vi "SLSC Convert Items - String to Variants.vi"(0 "Datatype":string, 5 "Value":string, 9 "Reset Value":string, 12 "enums":T1[](array[typedef]), 13 "string enums":cluster{"name":string, "string enums":string}[](array[cluster])) -> (4 "Value":variant, 6 "Reset Value":variant, 8 "Value (DBL)":dbl, 10 "Reset Value (DBL)":dbl)   [LabVIEW 2017, in "SLSC Tree Control.lvlib"]
doc: "Converts the string values of the tree control to variants and doubles datatypes."
uses:
  SLSC Tree Control.lvlib
  SLSC EDS API/JSON parsing/enum.ctl
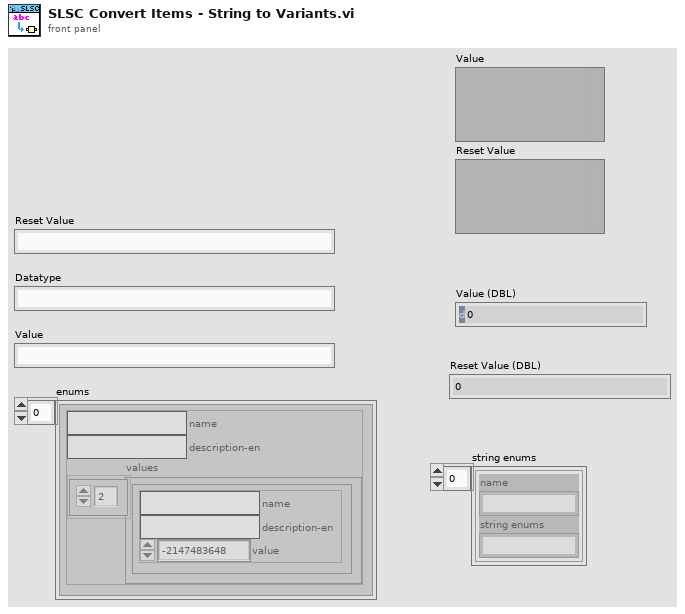
[diagram p1: front panel]
types:
  T1 = typedef "enum.ctl" = cluster{"name":string, "description-en":string, "values":cluster{"name":string, "description-en":string, "value":i32}[]}
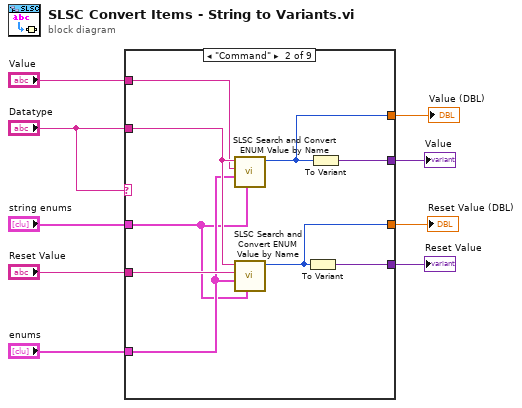
[diagram p0: block diagram]
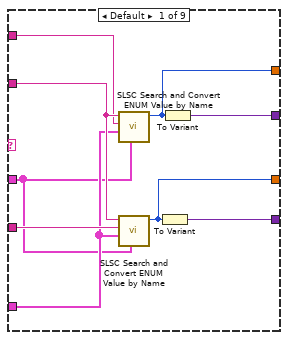
[diagram p2: hidden frame]
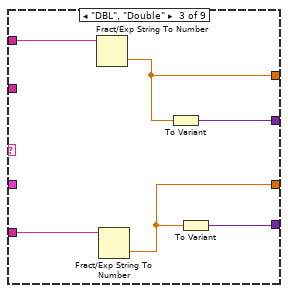
[diagram p3: hidden frame]
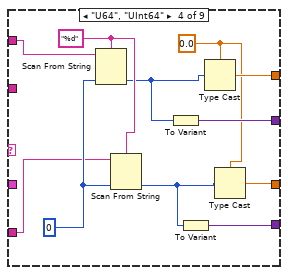
[diagram p4: hidden frame]
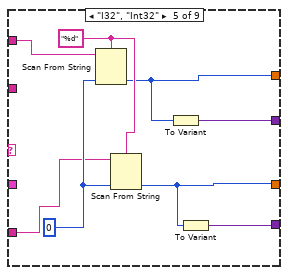
[diagram p5: hidden frame]
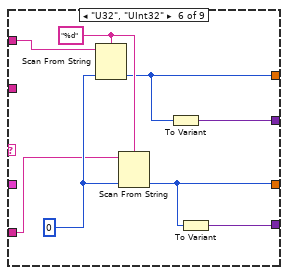
[diagram p6: hidden frame]
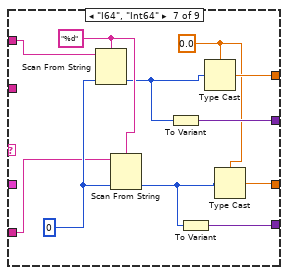
[diagram p7: hidden frame]
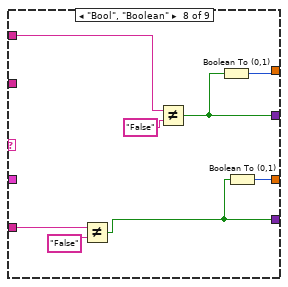
[diagram p8: hidden frame]
diagram:
  n1 = case shown="\"Command\"" "Datatype" {
    tunnel: "Reset Value" -> [w18 w27 w31 w40 w49 w56 w67 w77 _]
    tunnel: "Datatype" -> [w17 w26 _ _ _ _ _ _ _]
    tunnel: "enums" -> [w16 w25 _ _ _ _ _ _ _]
    tunnel: "string enums" -> [w15 w24 _ _ _ _ _ _ _]
    tunnel: "Value" -> [w14 w23 w32 w42 w45 w58 w69 w76 w80]
    tunnel: [w13 w22 w33 w44 w52 w60 w71 w74 w80] -> w4
    tunnel: [w12 w21 w30 w43 w51 w59 w70 w72 _] -> w3
    tunnel: [w11 w20 w29 w37 w47 w54 w64 w75 _] -> w2
    tunnel: [w10 w19 w28 w36 w46 w53 w63 w73 _] -> w1
    frame Default {
      n2 = call "SLSC Search and Convert ENUM Value by Name.vi"("Enum Strings"=w15, "enums"=w16, "Value"=w14, "Datatype Name"=w17) -> ("Value"=w11:i32)  [unwired: 5 in, 2 out]
      n3 = call "SLSC Search and Convert ENUM Value by Name.vi"("Enum Strings"=w15, "enums"=w16, "Value"=w18, "Datatype Name"=w17) -> ("Value"=w10:i32)  [unwired: 5 in, 2 out]
      n4 = To Variant(anything=w10) -> (Variant=w12:variant)
      n5 = To Variant(anything=w11) -> (Variant=w13:variant)
    }
    frame "Command" {
      n6 = call "SLSC Search and Convert ENUM Value by Name.vi"("Enum Strings"=w24, "enums"=w25, "Value"=w23, "Datatype Name"=w26) -> ("Value"=w20:i32)  [unwired: 5 in, 2 out]
      n7 = call "SLSC Search and Convert ENUM Value by Name.vi"("Enum Strings"=w24, "enums"=w25, "Value"=w27, "Datatype Name"=w26) -> ("Value"=w19:i32)  [unwired: 5 in, 2 out]
      n8 = To Variant(anything=w19) -> (Variant=w21:variant)
      n9 = To Variant(anything=w20) -> (Variant=w22:variant)
    }
    frame "DBL", "Double" {
      n10 = Fract/Exp String To Number(string=w32) -> (number=w29:dbl)  [unwired: 3 in, 1 out]
      n11 = Fract/Exp String To Number(string=w31) -> (number=w28:dbl)  [unwired: 3 in, 1 out]
      n12 = To Variant(anything=w29) -> (Variant=w33:variant)
      n13 = To Variant(anything=w28) -> (Variant=w30:variant)
    }
    frame "U64", "UInt64" {
      w34 = 0.0 ("Value")
      w39 = "%d" ("format string")
      w41 = u64 0 ("default (0 U32)")
      n14 = Scan From String(format string=w39, input string=w42, default 1=w41) -> (output 1=w38:u64)  [unwired: 2 in, 3 out]
      n15 = Scan From String(format string=w39, input string=w40, default 1=w41) -> (output 1=w35:u64)  [unwired: 2 in, 3 out]
      n16 = To Variant(anything=w38) -> (Variant=w44:variant)
      n17 = To Variant(anything=w35) -> (Variant=w43:variant)
      n18 = Type Cast(type=w34, x=w38) -> (*(type *) &x=w37:dbl)
      n19 = Type Cast(type=w34, x=w35) -> (*(type *) &x=w36:dbl)
    }
    frame "I32", "Int32" {
      w48 = "%d" ("format string")
      w50 = 0 ("default (0 U32)")
      n20 = Scan From String(format string=w48, input string=w45, default 1=w50) -> (output 1=w47:i32)  [unwired: 2 in, 3 out]
      n21 = Scan From String(format string=w48, input string=w49, default 1=w50) -> (output 1=w46:i32)  [unwired: 2 in, 3 out]
      n22 = To Variant(anything=w47) -> (Variant=w52:variant)
      n23 = To Variant(anything=w46) -> (Variant=w51:variant)
    }
    frame "U32", "UInt32" {
      w55 = "%d" ("format string")
      w57 = u32 0 ("default (0 U32)")
      n24 = Scan From String(format string=w55, input string=w58, default 1=w57) -> (output 1=w54:u32)  [unwired: 2 in, 3 out]
      n25 = Scan From String(format string=w55, input string=w56, default 1=w57) -> (output 1=w53:u32)  [unwired: 2 in, 3 out]
      n26 = To Variant(anything=w54) -> (Variant=w60:variant)
      n27 = To Variant(anything=w53) -> (Variant=w59:variant)
    }
    frame "I64", "Int64" {
      w61 = 0.0 ("Value")
      w66 = "%d" ("format string")
      w68 = i64 0 ("default (0 U32)")
      n28 = Scan From String(format string=w66, input string=w69, default 1=w68) -> (output 1=w65:i64)  [unwired: 2 in, 3 out]
      n29 = Scan From String(format string=w66, input string=w67, default 1=w68) -> (output 1=w62:i64)  [unwired: 2 in, 3 out]
      n30 = To Variant(anything=w65) -> (Variant=w71:variant)
      n31 = To Variant(anything=w62) -> (Variant=w70:variant)
      n32 = Type Cast(type=w61, x=w65) -> (*(type *) &x=w64:dbl)
      n33 = Type Cast(type=w61, x=w62) -> (*(type *) &x=w63:dbl)
    }
    frame "Bool", "Boolean" {
      n34 = Not Equal?(x=w77, y="False") -> (x != y?=w72:bool)
      n35 = Not Equal?(x=w76, y="False") -> (x != y?=w74:bool)
      n36 = Boolean To (0,1)(Boolean=w74) -> (0, 1=w75:i16)
      n37 = Boolean To (0,1)(Boolean=w72) -> (0, 1=w73:i16)
    }
    frame "String" {
    }
  }
  "Value" <- w4
  "Reset Value" <- w3
  "Value (DBL)" <- w2
  "Reset Value (DBL)" <- w1
